vi "军蚁-Initial Camera - 副本.vi"(8 "error in (no error)":errorcluster caption="错误输入（无错误）") -> (0 "error out":errorcluster caption="错误输出", 1 "cam1":T1, 2 "cam0":T1, 3 "Session Out":T1)   [LabVIEW 2017]
uses:
  <vilib>/userdefined/High Color/IMAQdx.ctl
  <vilib>/vision/driver/IMAQdx.llb/IMAQdx Camera Control Mode.ctl
  <vilib>/vision/driver/NI_Vision_Acquisition_Software.lvlib
  <vilib>/vision/driver/IMAQdx.llb/IMAQdx Acquisition Mode.ctl
  <resource>/objmgr/imaqdx.rc
panel:
  in  "曝光值":i64=500 caption="ValueI64" min=500 max=5000000
  out "数组":T1[](array[typedef])
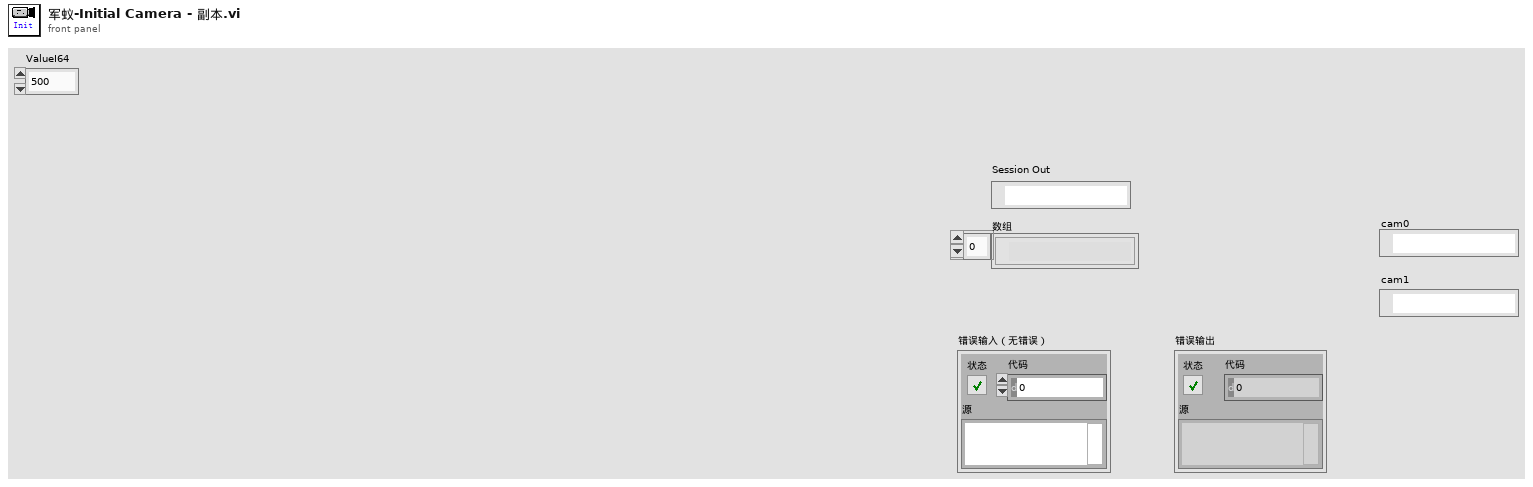
[diagram p1: front panel]
types:
  T1 = typedef "IMAQdx.ctl" = refnum<k21>
  T2 = typedef "NI_Vision_Acquisition_Software.lvlib/IMAQdx Camera Control Mode.ctl" = enum32{"Controller", "Listener"}
  T3 = typedef "NI_Vision_Acquisition_Software.lvlib/IMAQdx Acquisition Mode.ctl" = enum32{"One Shot", "Continuous"}
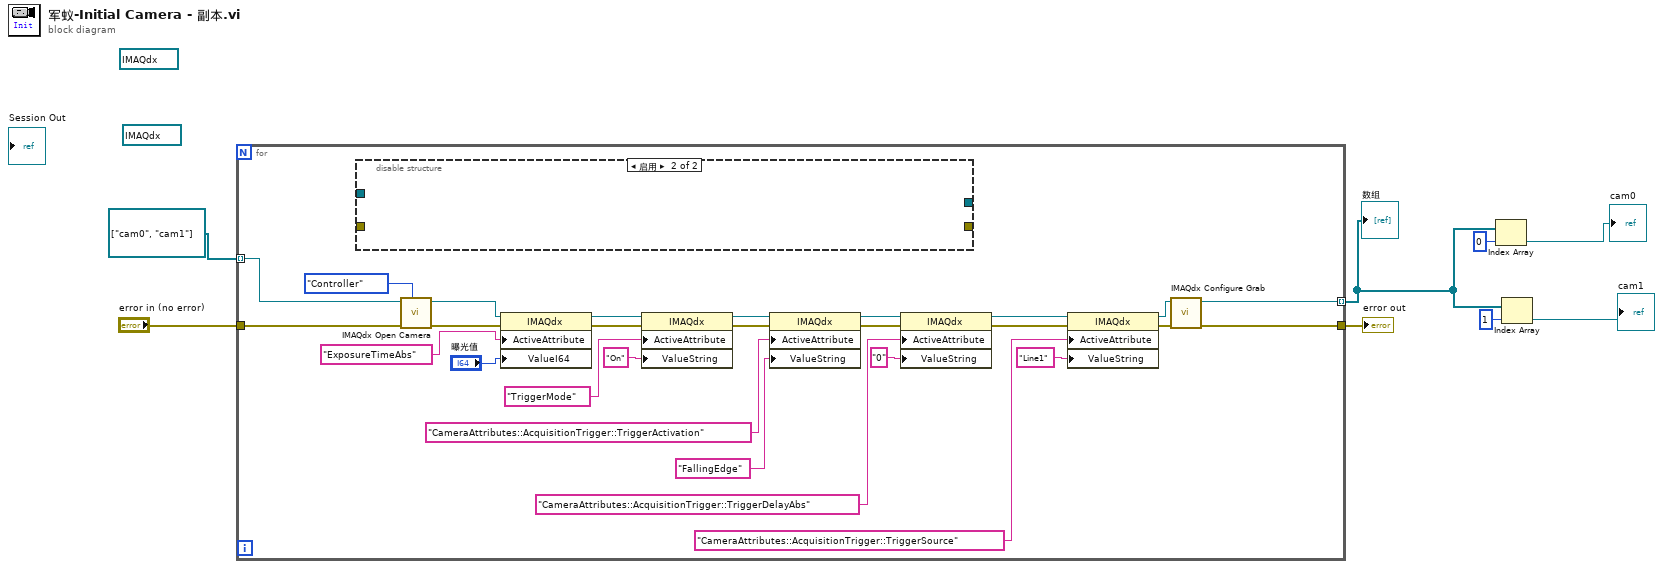
[diagram p0: block diagram]
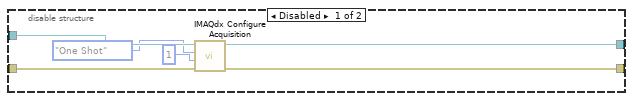
[diagram p2: hidden frame]
diagram:
  (unwired) T1 "cam0" ("Session Iin")
  (unwired) T1 "cam0" ("Session Iin")
  n1 = for {
    tunnel: "error in (no error)" -> [w35]
    tunnel: [w9] -> w7
    tunnel: T1[] ["cam0", "cam1"] -> [w33] mode=indexing
    tunnel: [w10] -> w3 mode=indexing
    n2 = disable-structure shown="启用" {
      disable-tunnel: [w41 _] -> _
      disable-tunnel: _ -> [w40 _]
      disable-tunnel: _ -> [w37 _]
      disable-tunnel: [w36 _] -> _
      frame Disabled {
        n3 = call <vilib>:"IMAQdx Configure Acquisition.vi"("error in"=w37, "Number of Buffers"=u32 1, "Continuous?"=IMAQdx_Acquisition_Mode."One Shot", "Session In"=w40) -> ("error out"=w41:errorcluster, "Session Out"=w36:T1)  [unwired: 6 in]
      }
      frame Enabled {
      }
    }
    n4 = call <vilib>:"IMAQdx Open Camera.vi"("Camera Control Mode"=IMAQdx_Camera_Control_Mode."Controller", "error in"=w35, "Session In"=w33) -> ("error out"=w25:errorcluster, "Session Out"=w26:T1)  [unwired: 7 in]
    n5 = property class="IMAQdx"(reference=w26, error in=w25, "ActiveAttribute"="ExposureTimeAbs", "ValueI64"="曝光值") -> (reference out=w32:T1, error out=w31:errorcluster)
    n6 = property class="IMAQdx"(reference=w32, error in=w31, "ActiveAttribute"="TriggerMode", "ValueString"="On") -> (reference out=w29:T1, error out=w30:errorcluster)
    n7 = property class="IMAQdx"(reference=w29, error in=w30, "ActiveAttribute"="CameraAttributes::AcquisitionTrigger::TriggerActivation", "ValueString"="FallingEdge") -> (reference out=w20:T1, error out=w19:errorcluster)
    n8 = property class="IMAQdx"(reference=w20, error in=w19, "ActiveAttribute"="CameraAttributes::AcquisitionTrigger::TriggerDelayAbs", "ValueString"="0") -> (reference out=w22:T1, error out=w21:errorcluster)
    n9 = property class="IMAQdx"(reference=w22, error in=w21, "ActiveAttribute"="CameraAttributes::AcquisitionTrigger::TriggerSource", "ValueString"="Line1") -> (reference out=w23:T1, error out=w24:errorcluster)
    n10 = call <vilib>:"IMAQdx Configure Grab.vi"("error in"=w24, "Session In"=w23) -> ("error out"=w9:errorcluster, "Session Out"=w10:T1)  [unwired: 8 in]
  }
  "error out" <- w7
  "数组" <- w3
  n11 = Index Array(array=w3, index=0 ("索引")) -> (element=→"cam0":T1)
  n12 = Index Array(array=w3, index=1 ("索引")) -> (element=→"cam1":T1)
